vi "random bullet.vi"(7 "chamber capacity":u32) -> (1 "empty rounds":u32, 2 "live rounds":u32)   [LabVIEW 2025]
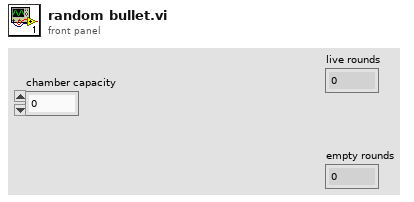
[diagram p1: front panel]
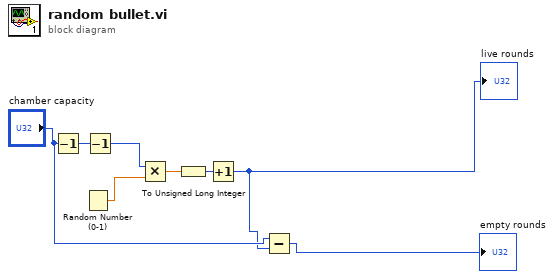
[diagram p0: block diagram]
diagram:
  n1 = Decrement(x="chamber capacity") -> (x-1=w5:u32)
  n2 = Random Number (0-1)() -> (number: 0 to 1=w8:dbl)
  n3 = Decrement(x=w5) -> (x-1=w4:u32)
  n4 = Multiply(x=w4, y=w8) -> (x*y=w7:dbl)
  n5 = To Unsigned Long Integer(number=w7) -> (unsigned 32bit integer=w6:u32)
  n6 = Increment(x=w6) -> (x+1=w2:u32)
  "live rounds" <- w2
  n7 = Subtract(x="chamber capacity", y=w2) -> (x-y=→"empty rounds":u32)
